vi "ReadTemplateSettings.vi"(10 "CommonClassTemplate":bool, 11 "TemplateFolder":path) -> (3 "TemplateSettings":T1)   [LabVIEW 2012, in "ClassWriterNative.lvclass"]
uses:
  <resource>/Framework/Providers/Open_GDS/ClassProviders/Provider_LvNativeClass/ClassWriterNative_class/ClassWriterNative.lvclass
  <resource>/Framework/Providers/Open_GDS/ClassProviders/Provider_BaseClassInterface/ClassWriter_class/TemplateSettings.ctl
  <vilib>/Utility/config.llb/Read Key (Boolean).vi
  <resource>/Framework/Providers/Open_GDS/ClassProviders/Provider_BaseClassInterface/ClassWriter_class/ClassWriter.lvclass
  <vilib>/Utility/config.llb/NI_LVConfig.lvlib
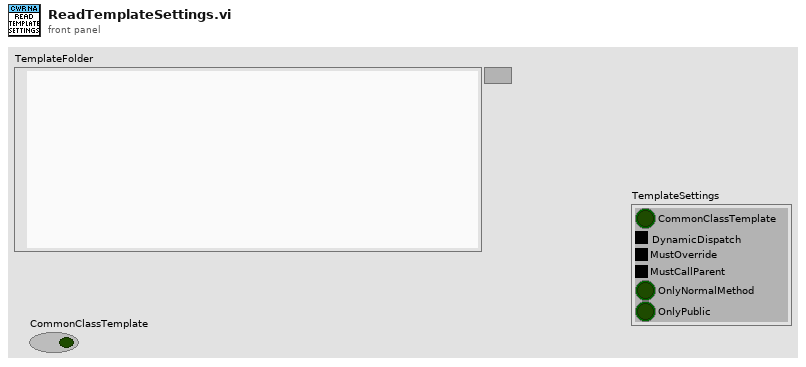
[diagram p1: front panel]
types:
  T1 = typedef "ClassWriter.lvclass/TemplateSettings.ctl" = cluster{"CommonClassTemplate":bool, "DynamicDispatch":enum8{"False", "True", "Mixed"}, "MustOverride":enum8{"False", "True", "Mixed"}, "MustCallParent":enum8{"False", "True", "Mixed"}, "OnlyNormalMethod":bool, "OnlyPublic":bool}
  T2 = typedef "NI_LVConfig.lvlib/Config Data RefNum.ctl" = refnum<k1>
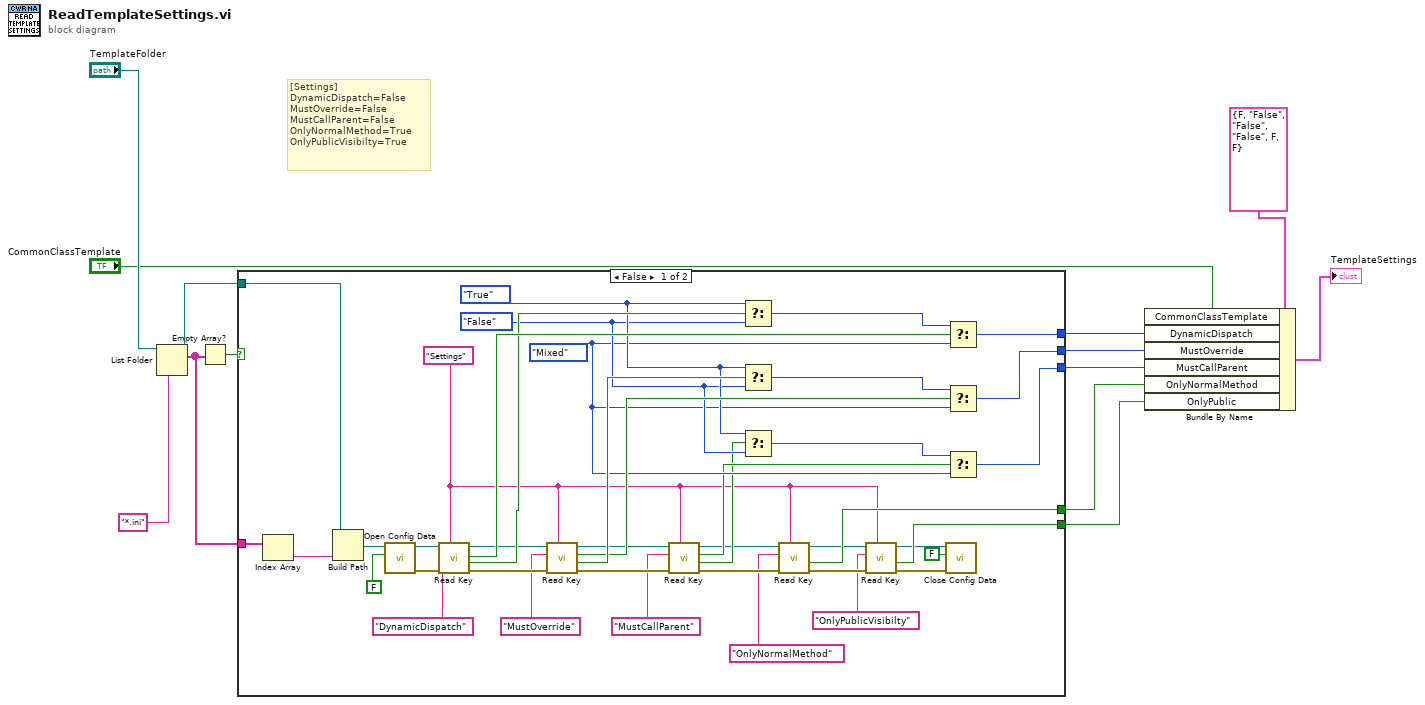
[diagram p0: block diagram]
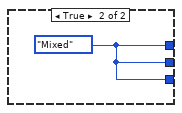
[diagram p2: hidden frame]
diagram:
  # "[Settings]\nDynamicDispatch=False\nMustOverride=False\nMustCallParent=False\nOnlyNormalMethod=True\nOnlyPublicVisibilty=True"
  n1 = List Folder(path="TemplateFolder", pattern="*.ini") -> (path out=w13:path, filenames=w12:string[])  [unwired: 2 in, 2 out]
  n2 = Empty Array?(array=w12) -> (empty?=w11:bool)
  n3 = case shown="False" w11 {
    tunnel: w12 -> [w54 _]
    tunnel: w13 -> [w52 _]
    tunnel: [w42 w55] -> w5
    tunnel: [w32 w55] -> w4
    tunnel: [w25 w55] -> w3
    tunnel: [w22 _] -> w2
    tunnel: [w17 _] -> w1
    frame False {
      w29 = enum8{"False", "True", "Mixed"}."False" ("DynamicDispatch")
      w30 = enum8{"False", "True", "Mixed"}."True" ("DynamicDispatch")
      w28 = enum8{"False", "True", "Mixed"}."Mixed" ("DynamicDispatch")
      w14 = "Settings" ("section")
      n4 = Index Array(array=w54) -> (element=w53:string)  [unwired: 1 in]
      n5 = Build Path(base path=w52, name or relative path=w53) -> (appended path=w51:path)
      n6 = call <vilib>:"Open Config Data.vi"("create file if necessary (T)"=FALSE, "configuration file path"=w51) -> ("error out"=w49:errorcluster, "refnum"=w50:T2)  [unwired: 7 in, 1 out]
      n7 = call-poly <vilib>:"Read Key.vi"("section"=w14, "error in (no error)"=w49, "key"="DynamicDispatch", "refnum"=w50) -> ("error out"=w40:errorcluster, "value"=w44:bool, "found?"=w46:bool, "refnum out"=w41:T2)  [unwired: 4 in]
      n8 = call-poly <vilib>:"Read Key.vi"("section"=w14, "error in (no error)"=w40, "key"="MustOverride", "refnum"=w41) -> ("error out"=w34:errorcluster, "value"=w37:bool, "found?"=w36:bool, "refnum out"=w35:T2)  [unwired: 4 in]
      n9 = call-poly <vilib>:"Read Key.vi"("section"=w14, "error in (no error)"=w34, "key"="MustCallParent", "refnum"=w35) -> ("error out"=w23:errorcluster, "value"=w26:bool, "found?"=w27:bool, "refnum out"=w24:T2)  [unwired: 4 in]
      n10 = Select(t=w30, s=w44, f=w29) -> (s? t:f=w43:enum8{"False", "True", "Mixed"})
      n11 = Select(t=w30, s=w37, f=w29) -> (s? t:f=w38:enum8{"False", "True", "Mixed"})
      n12 = Select(t=w30, s=w26, f=w29) -> (s? t:f=w31:enum8{"False", "True", "Mixed"})
      n13 = call-poly <vilib>:"Read Key.vi"("section"=w14, "error in (no error)"=w23, "key"="OnlyNormalMethod", "refnum"=w24) -> ("error out"=w19:errorcluster, "value"=w22:bool, "refnum out"=w20:T2)  [unwired: 4 in, 1 out]
      n14 = call-poly <vilib>:"Read Key.vi"("section"=w14, "error in (no error)"=w19, "key"="OnlyPublicVisibilty", "refnum"=w20) -> ("error out"=w15:errorcluster, "value"=w17:bool, "refnum out"=w16:T2)  [unwired: 4 in, 1 out]
      n15 = call <vilib>:"Close Config Data.vi"("error in (no error)"=w15, "write file if changed (T)"=FALSE, "refnum"=w16) -> ()  [unwired: 7 in, 2 out]
      n16 = Select(t=w43, s=w46, f=w28) -> (s? t:f=w42:enum8{"False", "True", "Mixed"})
      n17 = Select(t=w38, s=w36, f=w28) -> (s? t:f=w32:enum8{"False", "True", "Mixed"})
      n18 = Select(t=w31, s=w27, f=w28) -> (s? t:f=w25:enum8{"False", "True", "Mixed"})
    }
    frame True {
      w55 = enum8{"False", "True", "Mixed"}."Mixed" ("DynamicDispatch")
    }
  }
  n19 = Bundle By Name(cluster=T1 {"CommonClassTemplate"=FALSE, "DynamicDispatch"=enum."False", "MustOverride"=enum."False", "MustCallParent"=enum."False", "OnlyNormalMethod"=FALSE, "OnlyPublic"=FALSE} ("TemplateSettings"), "CommonClassTemplate"="CommonClassTemplate", "DynamicDispatch"=w5, "MustOverride"=w4, "MustCallParent"=w3, "OnlyNormalMethod"=w2, "OnlyPublic"=w1) -> (→"TemplateSettings":T1)
